vi "Get Selected Profile from List.vi"(8 "Fehler (Eingang, kein Fehler)":errorcluster, 11 "Referenz":refnum<vi>) -> (0 "error out":errorcluster, 3 "Selected Profile Path":path)   [LabVIEW 2016, in "Scan Engine Custom Device.lvlib"]
uses:
  Scan Engine Custom Device.lvlib
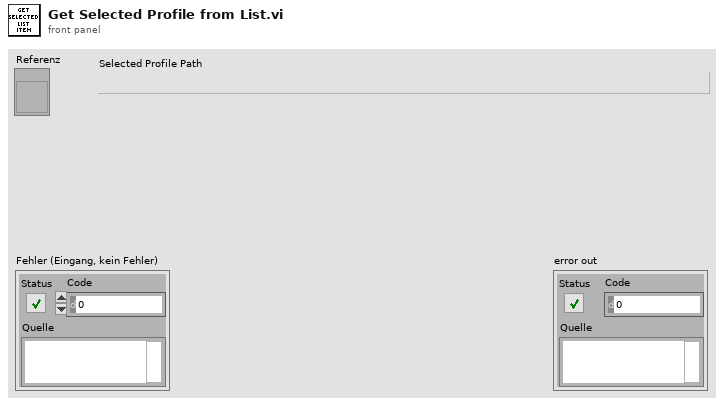
[diagram p1: front panel]
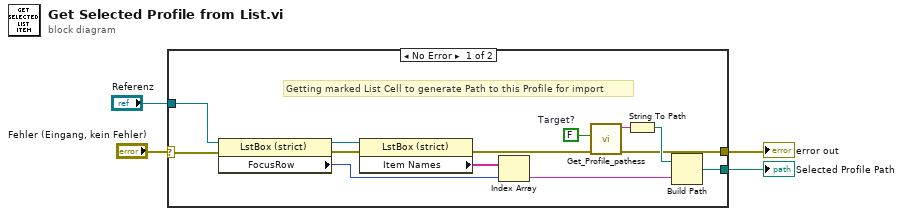
[diagram p0: block diagram]
diagram:
  n1 = case shown="No Error" "Fehler (Eingang, kein Fehler)" {
    selector: "Fehler (Eingang, kein Fehler)" -> [w8 w18]
    tunnel: "Referenz" -> [w7 _]
    tunnel: [w6 w18] -> w1
    tunnel: [w5 _] -> w2
    frame No Error {
      w13 = FALSE  # Target?
      # "Getting marked List Cell to generate Path to this Profile for import"
      n2 = property on="Property Node" class="LstBox (strict)"(reference=w7, error in=w8) -> (reference out=w9:refnum<vi>, error out=w10:errorcluster, "FocusRow"=w12:i32)
      n3 = property on="Property Node" class="LstBox (strict)"(reference=w9, error in=w10) -> (error out=w17:errorcluster, "Item Names"=w11:string[])  [unwired: 1 out]
      n4 = Index Array(array=w11, index=w12) -> (element=w16:string)
      n5 = call "Get_Profile_pathess.vi"("error in (no error)"=w17, "Target?"=w13) -> ("error out"=w6:errorcluster, "profileDestPath"=w14:string)  [unwired: 8 in]
      n6 = String To Path(string=w14) -> (path=w15:path)
      n7 = Build Path(base path=w15, name or relative path=w16) -> (appended path=w5:path)
    }
    frame Error {
    }
  }
  "Selected Profile Path" <- w2
  "error out" <- w1
